vi "PH_Cont-601k_PSU.Set safe State.vi"(0 "VI in":refnum<vi>, 5 "error in (no error)":errorcluster) -> (14 "VI out":refnum<vi>, 19 "error out":errorcluster)   [LabVIEW 2014, in "PH_Cont-601k_PSU.lvlib"]
doc: "Whithin this VI the device specific own attributes are set to safe values and the readyness is recalculated. No talk to device is done."
uses:
  PH_Cont-601k_PSU.lvlib
  PH_Cont-601k_PSU.Configuration.ctl
  PH_Cont-601k_PSU.Mode.ctl
  PH_Cont-601k_PSU.Readyness Device.ctl
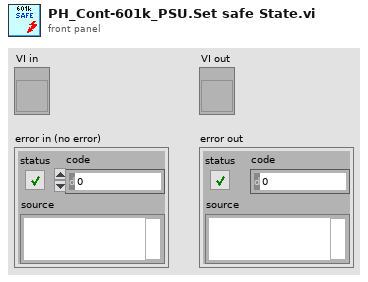
[diagram p1: front panel]
types:
  T1 = typedef "PH_Cont-601k_PSU.lvlib/PH_Cont-601k_PSU.Readyness Device.ctl" = enum32{"OFF", "CONNECTING", "CONNECTED", "OPERATING", "EOC", "ERROR"}
  T2 = typedef "PH_Cont-601k_PSU.lvlib/PH_Cont-601k_PSU.Mode.ctl" = enum32{"STOP", "STANDBY", "READY", "EMISSION", "ERROR"}
  T3 = typedef "PH_Cont-601k_PSU.lvlib/PH_Cont-601k_PSU.Configuration.ctl" = u16
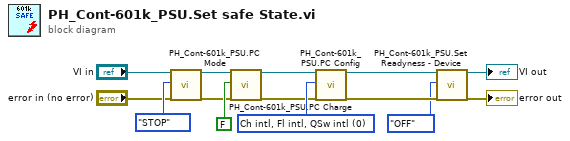
[diagram p0: block diagram]
diagram:
  w13 = T3 0 items=["Ch intl, Fl intl, QSw intl", "Ch intl, Fl intl, QSw ext", "Ch intl, Fl ext, QSw intl", "Ch intl, Fl ext, QSw ext", "Ch ext, Fl int, QSw int", "Ch ext, Fl int, QSw ext", "Ch ext, Fl ext, QSw int", "Ch ext, Fl ext, QSw ext"] ("Configuration")
  n1 = call "PH_Cont-601k_PSU.PC Mode.vi"("VI in"="VI in", "Mode"=PH_Cont-601k_PSU.Mode."STOP", "error in (no error)"="error in (no error)") -> ("VI out"=w9:refnum<vi>, "error out"=w8:errorcluster)  [unwired: 14 in, 1 out]
  n2 = call "PH_Cont-601k_PSU.PC Charge.vi"("VI in"=w9, "Charge"=FALSE ("Configuration changed?"), "error in (no error)"=w8) -> ("VI out"=w2:refnum<vi>, "error out"=w1:errorcluster)  [unwired: 14 in, 1 out]
  n3 = call "PH_Cont-601k_PSU.PC Config.vi"("VI in"=w2, "Configuration"=w13, "error in (no error)"=w1) -> ("VI out"=w5:refnum<vi>, "error out"=w4:errorcluster)  [unwired: 14 in, 1 out]
  n4 = call "PH_Cont-601k_PSU.Set Readyness - Device.vi"("VI in"=w5, "Readyness - Device"=PH_Cont-601k_PSU.Readyness_Device."OFF" ("Readyness.Device"), "error in (no error)"=w4) -> ("VI out"=→"VI out":refnum<vi>, "error out"=→"error out":errorcluster)  [unwired: 15 in]
